vi "GLBL_AO_9265.vi"(10 "AO_0_3":T1, 11 "write_read":bool) -> (2 "AO_0_3 out":T1)   [LabVIEW 2020]
uses:
  MPB/IO/controls/AO_0_3.ctl
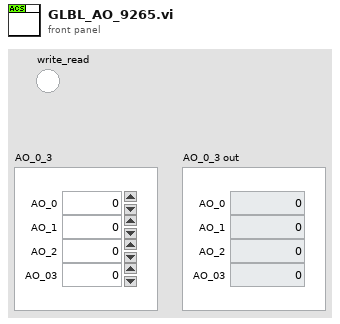
[diagram p1: front panel]
types:
  T1 = typedef "AO_0_3.ctl" = cluster{"AO_0":dbl, "AO_1":dbl, "AO_2":dbl, "AO_03":dbl}
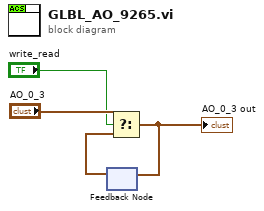
[diagram p0: block diagram]
diagram:
  n1 = feedback #1() -> (w3:T1)  [unwired: 1 in]
  n2 = Select(t="AO_0_3", s="write_read", f=w3) -> (s? t:f=w2:T1)
  "AO_0_3 out" <- w2
  n3 = feedback-in #1(w2) -> ()
